vi "主程序.vi"() -> ()   [LabVIEW 2018]
panel:
  out "总用时（s）":dbl
  out "结束时间":u32
  out "开始时间":u32
  out "错误输出":errorcluster
  out "sigma大小5":i32[](array[numeric])
  out "sigma大小4":i32[](array[numeric])
  out "sigma大小3":i32[](array[numeric])
  out "sigma大小2":i32[](array[numeric])
  out "sigma大小1":i32[](array[numeric])
  out "sigma大小":i32[](array[numeric])
  out "cof大小":i32[](array[numeric])
  out "识别结束":bool
  out "最大值":i32
  out "距离":dbl[](array[numeric])
  out "训练完成":bool
  in  "说话人 6 sigma 2":path=path "D:/Desktop/audio/sigma_anjiale3.lvm"
  in  "说话人 6 mu 2":path=path "D:/Desktop/audio/mu_anjiale3.lvm"
  in  "说话人 5 sigma 2":path=path "D:/Desktop/audio/sigma_zhuqiseng3.lvm"
  in  "说话人 5 mu 2":path=path "D:/Desktop/audio/mu_zhuqiseng3.lvm"
  in  "说话人 4 sigma 2":path=path "D:/Desktop/audio/sigma_lianglv3.lvm"
  in  "说话人 4 mu 2":path=path "D:/Desktop/audio/mu_lianglv3.lvm"
  in  "说话人 4 pai 2":path=path "D:/Desktop/audio/pai_lianglv3.lvm"
  in  "说话人 3 sigma 2":path=path "D:/Desktop/audio/sigma_叶雪花.lvm"
  in  "说话人 3 mu 2":path=path "D:/Desktop/audio/mu_叶雪花.lvm"
  in  "说话人 3 pai 2":path=path "D:/Desktop/audio/pai_叶雪花.lvm"
  in  "说话人 2 sigma 2":path=path "D:/Desktop/audio/sigma_赵霞.lvm"
  in  "说话人 2 mu 2":path=path "D:/Desktop/audio/mu_赵霞.lvm"
  in  "说话人 2 pai 2":path=path "D:/Desktop/audio/pai_赵霞.lvm"
  in  "说话人 1 sigma":path=path "D:/Desktop/audio/sigma_胡楠.lvm"
  in  "说话人 1 mu":path=path "D:/Desktop/audio/mu_胡楠.lvm"
  out "提示框":string
  out "滤波后":dbl[](graph)
  out "待识别语音":dbl[](graph)
  in  "说话人 6 pai":path=path "D:/Desktop/audio/pai_anjiale3.lvm"
  in  "说话人 5 pai":path=path "D:/Desktop/audio/pai_zhuqiseng3.lvm"
  in  "说话人 1 pai":path=path "D:/Desktop/audio/pai_胡楠.lvm"
  out "确定的人":string
  out "最大似然距离":dbl format="%.2f"
  in  "语音识别":bool
  in  "语音训练":bool
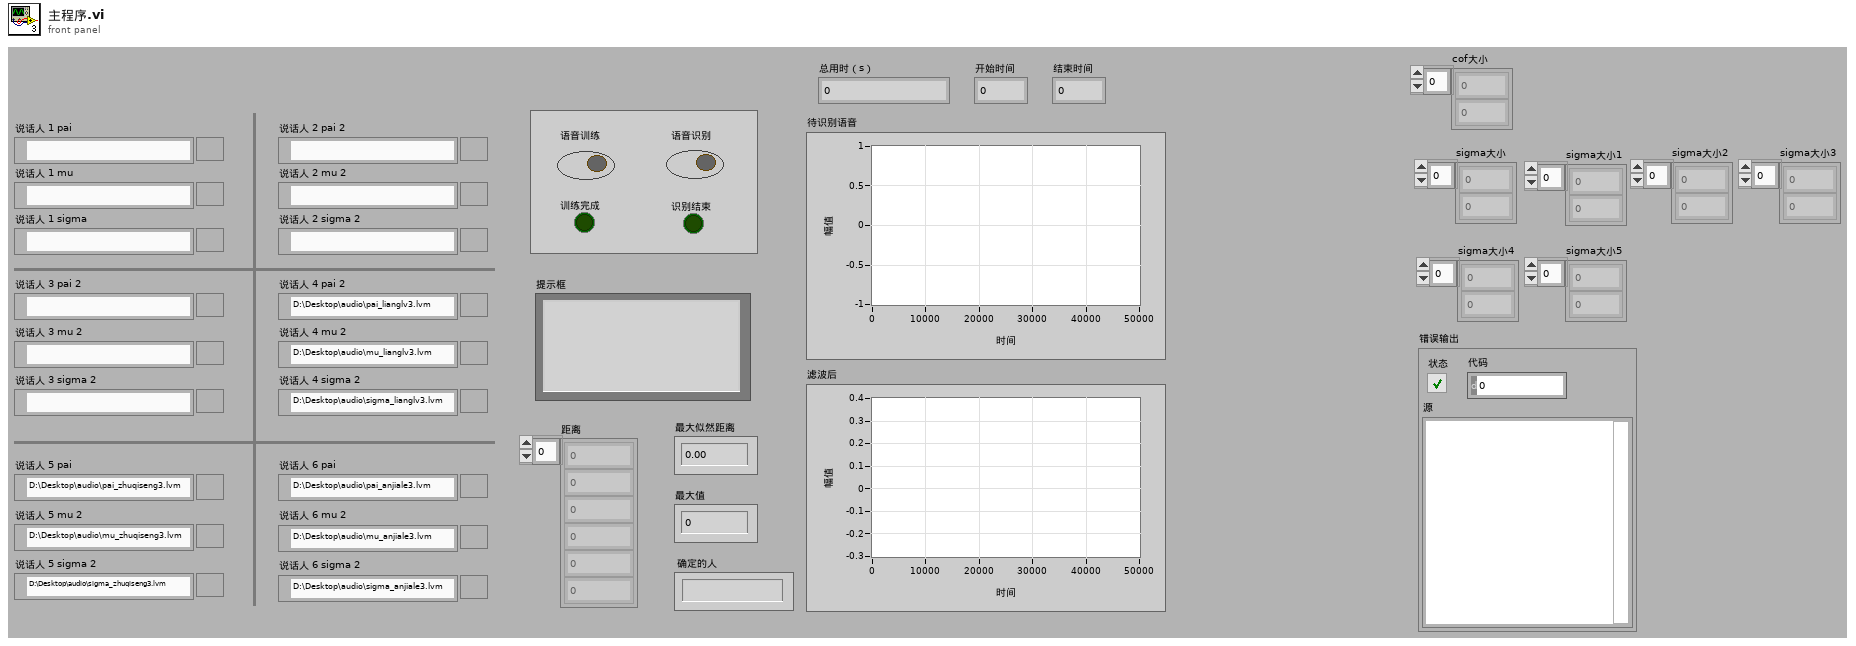
[diagram p1: front panel]
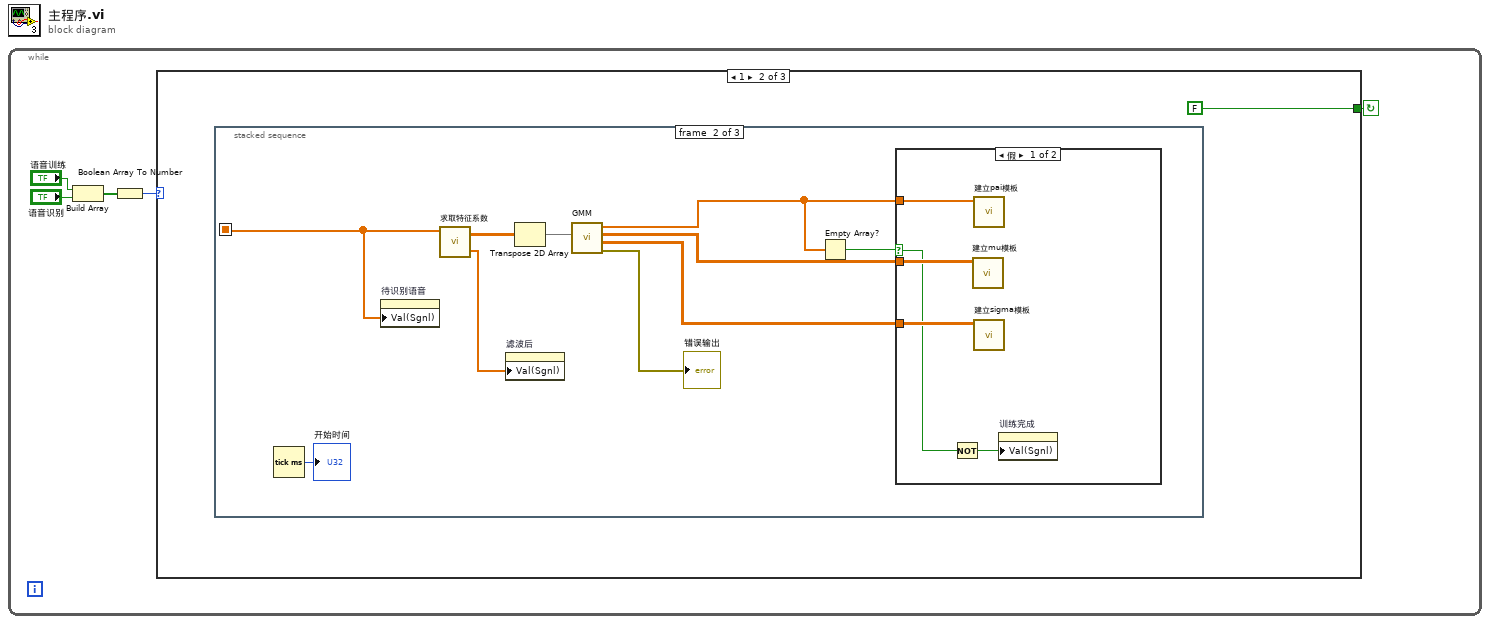
[diagram p0: block diagram]
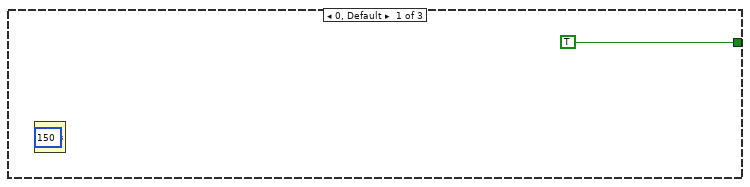
[diagram p2: hidden frame]
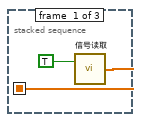
[diagram p3: hidden frame]
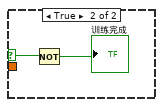
[diagram p4: hidden frame]
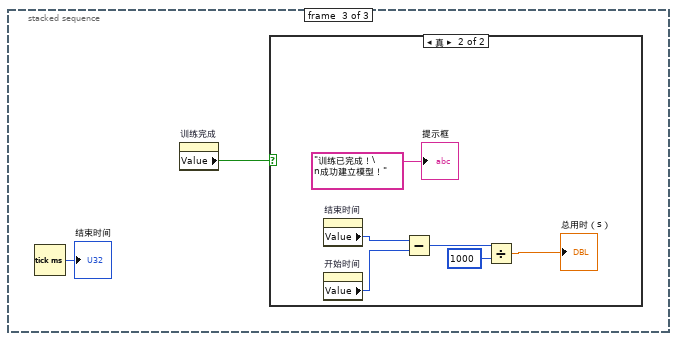
[diagram p5: hidden frame]
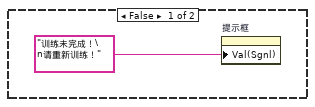
[diagram p6: hidden frame]
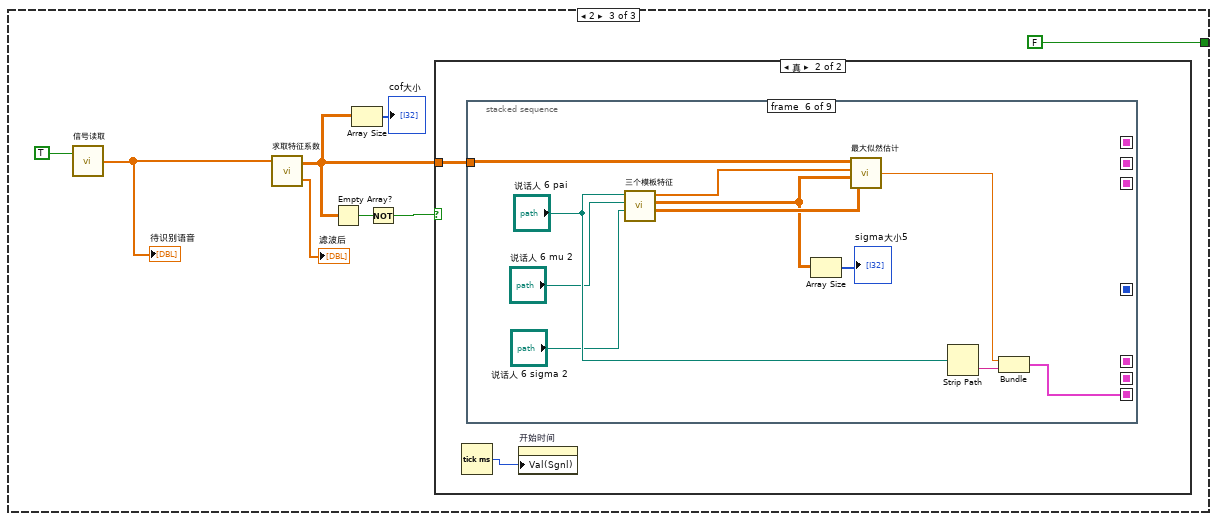
[diagram p7: hidden frame]
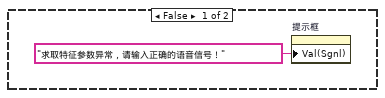
[diagram p8: hidden frame]
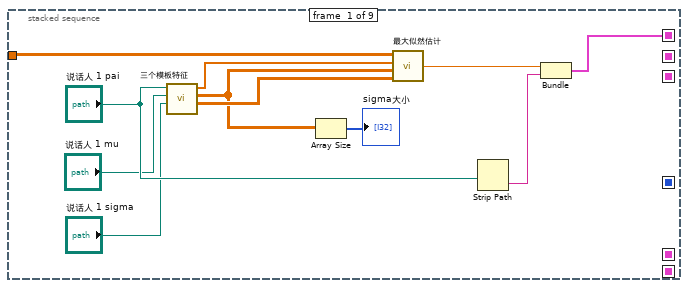
[diagram p9: hidden frame]
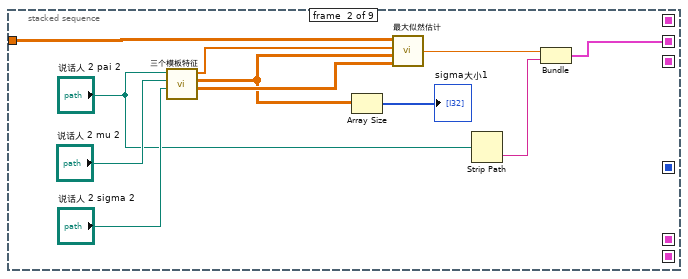
[diagram p10: hidden frame]
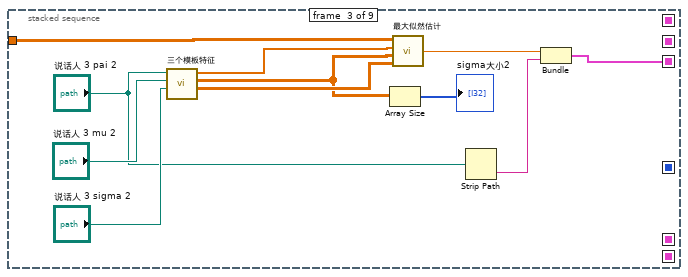
[diagram p11: hidden frame]
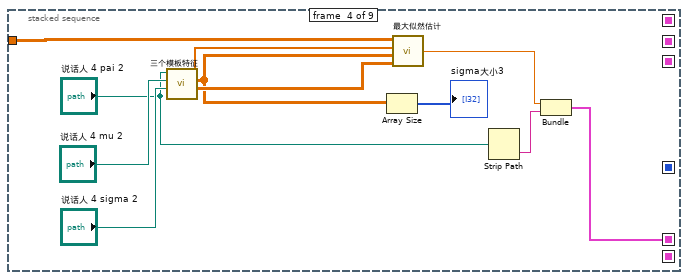
[diagram p12: hidden frame]
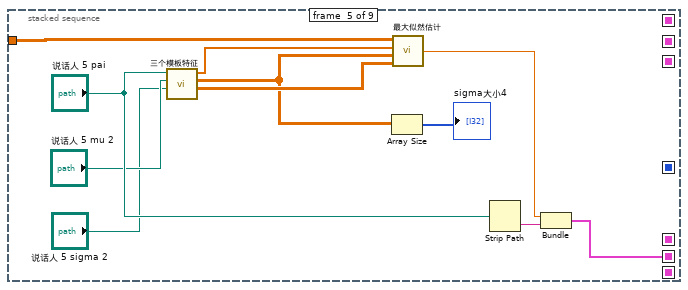
[diagram p13: hidden frame]
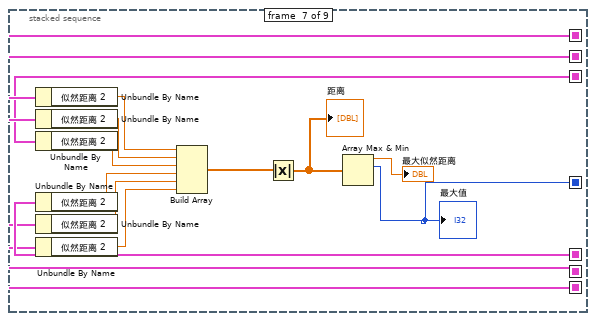
[diagram p14: hidden frame]
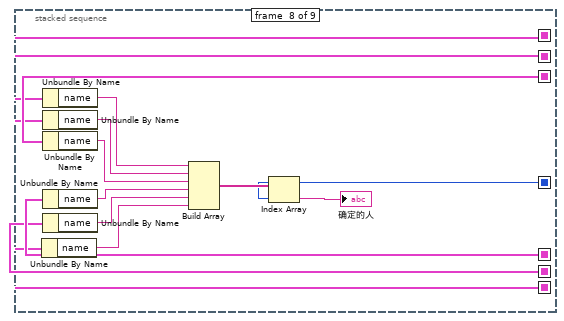
[diagram p15: hidden frame]
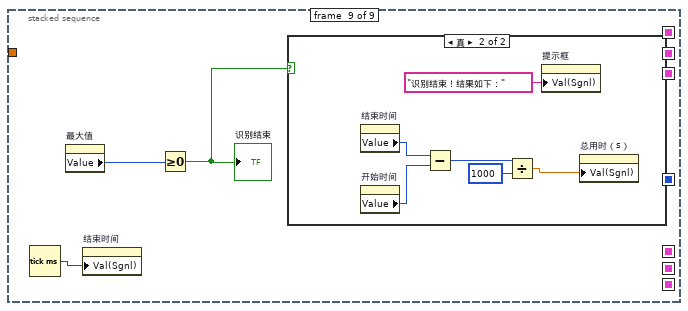
[diagram p16: hidden frame]
diagram:
  n1 = while {
    stop <- w1 continue-if-true
    n2 = Build Array("语音训练", "语音识别") -> (w3:bool[])
    n3 = Boolean Array To Number(Boolean array=w3) -> (number=w2:u32)
    n4 = case shown="1" w2 {
      tunnel: [TRUE FALSE FALSE] -> w1
      frame 0, Default {
        n5 = Wait (ms)(milliseconds to wait=u32 150) -> ()  [unwired: 1 out]
      }
      frame 1 {
        n6 = stacked-sequence {
          seq-local: [w9 _ _] -> [_ w11 _]
          frame #0 {
            n7 = call "信号读取.vi"("Boolean"=TRUE) -> ("mono 16-bit"=w9:dbl[])  [unwired: 1 in]
          }
          frame #1 {
            n8 = Tick Count (ms)() -> (millisecond timer value=→"开始时间":u32)
            n9 = property on="待识别语音" class="WFGraph (严格)"("Val(Sgnl)"=w11) -> ()  [unwired: 2 in, 2 out]
            n10 = call "求取特征系数.vi"("speech"=w11) -> ("波形图"=w16:dbl[], "cof"=w13:dbl[][])  [unwired: 2 in]
            n11 = property on="滤波后" class="WFGraph (严格)"("Val(Sgnl)"=w16) -> ()  [unwired: 2 in, 2 out]
            n12 = Transpose 2D Array(2D array=w13) -> (transposed array=w14:dbl[][])
            n13 = call "GMM.vi"("cof"=w14) -> ("错误输出"=→"错误输出":errorcluster, "sigema"=w20:dbl[][], "mu"=w19:dbl[][], "pai"=w17:dbl[])  [unwired: 6 in]
            n14 = Empty Array?(array=w17) -> (empty?=w18:bool)
            n15 = case shown="假" w18 {
              selector: w18 -> [w22 w27]
              tunnel: w17 -> [w25 _]
              tunnel: w19 -> [w24 _]
              tunnel: w20 -> [w23 _]
              frame False {
                n16 = Not(x=w22) -> (.not. x?=w21:bool)
                n17 = call "建立mu模板.vi"("输入MFCC"=w24) -> ()  [unwired: 11 in]
                n18 = call "建立pai模板.vi"("输入MFCC"=w25) -> ()  [unwired: 11 in]
                n19 = call "建立sigma模板.vi"("输入MFCC"=w23) -> ()  [unwired: 11 in]
                n20 = property on="训练完成" class="Bool (严格)"("Val(Sgnl)"=w21) -> ()  [unwired: 2 in, 2 out]
              }
              frame True {
                n21 = Not(x=w27) -> (.not. x?=→"训练完成":bool)
              }
            }
          }
          frame #2 {
            n22 = Tick Count (ms)() -> (millisecond timer value=→"结束时间":u32)
            n23 = property on="训练完成" class="Bool (严格)"() -> ("Value"=w29:bool)  [unwired: 2 in, 2 out]
            n24 = case shown="真" w29 {
              frame False {
                n25 = property on="提示框" class="Str"("Val(Sgnl)"="训练未完成！\n请重新训练！") -> ()  [unwired: 2 in, 2 out]
              }
              frame True {
                n26 = property on="结束时间" class="DigNum (严格)"() -> ("Value"=w32:u32)  [unwired: 2 in, 2 out]
                n27 = property on="开始时间" class="DigNum (严格)"() -> ("Value"=w31:u32)  [unwired: 2 in, 2 out]
                n28 = Subtract(x=w32, y=w31) -> (x-y=w34:u32)
                n29 = Divide(x=w34, y=u32 1000) -> (x/y=→"总用时（s）":dbl)
                "提示框" <- "训练已完成！\n成功建立模型！"
              }
            }
          }
        }
      }
      frame 2 {
        n30 = call "信号读取.vi"("Boolean"=TRUE) -> ("mono 16-bit"=w39:dbl[])  [unwired: 1 in]
        "待识别语音" <- w39
        n31 = call "求取特征系数.vi"("speech"=w39) -> ("波形图"=→"滤波后":dbl[], "cof"=w38:dbl[][])  [unwired: 2 in]
        n32 = Empty Array?(array=w38) -> (empty?=w43:bool)
        n33 = Array Size(array=w38) -> (size(s)=→"cof大小":i32[])
        n34 = Not(x=w43) -> (.not. x?=w42:bool)
        n35 = case shown="真" w42 {
          tunnel: w38 -> [_ w47]
          frame False {
            n36 = property on="提示框" class="Str"("Val(Sgnl)"="求取特征参数异常，请输入正确的语音信号！" ("值(信号)")) -> ()  [unwired: 2 in, 2 out]
          }
          frame True {
            n37 = Tick Count (ms)() -> (millisecond timer value=w46:u32)
            n38 = stacked-sequence {
              seq-local: [_ _ _ _ _ _ w115 _ _] -> [_ _ _ _ _ _ _ w137 _]
              seq-local: [w57 _ _ _ _ _ _ _ _] -> [_ _ _ _ _ _ w129 w134 _]
              seq-local: [_ w68 _ _ _ _ _ _ _] -> [_ _ _ _ _ _ w128 w135 _]
              seq-local: [_ _ w79 _ _ _ _ _ _] -> [_ _ _ _ _ _ w127 w136 _]
              seq-local: [_ _ _ w90 _ _ _ _ _] -> [_ _ _ _ _ _ w126 w133 _]
              seq-local: [_ _ _ _ w101 _ _ _ _] -> [_ _ _ _ _ _ w125 w132 _]
              seq-local: [_ _ _ _ _ w112 _ _ _] -> [_ _ _ _ _ _ w124 w131 _]
              tunnel: w47 -> [w51 w65 w77 w88 w98 w109 _ _ _]
              frame #0 {
                n39 = call "三个模板特征.vi"("Filename 3"="说话人 1 sigma", "Filename 2"="说话人 1 mu", "Filename"="说话人 1 pai") -> ("sigma 4"=w49:dbl[][], "mu 3"=w48:dbl[][], "pai 2"=w54:dbl[])  [unwired: 5 in]
                n40 = Array Size(array=w48) -> (size(s)=→"sigma大小":i32[])
                n41 = call "最大似然估计.vi"("sigma"=w49, "mu"=w48, "pai"=w54, "cof"=w51) -> ("似然距离 2"=w55:dbl)
                n42 = Strip Path(path="说话人 1 pai") -> (name=w58:string)  [unwired: 1 out]
                n43 = Bundle("似然距离 2"=w55, "name"=w58) -> (w57:cluster{"似然距离 2":dbl, "name":string})  [unwired: 1 in]
              }
              frame #1 {
                n44 = call "三个模板特征.vi"("Filename 3"="说话人 2 sigma 2", "Filename 2"="说话人 2 mu 2", "Filename"="说话人 2 pai 2") -> ("sigma 4"=w61:dbl[][], "mu 3"=w59:dbl[][], "pai 2"=w67:dbl[])  [unwired: 5 in]
                n45 = Array Size(array=w59) -> (size(s)=→"sigma大小1":i32[])
                n46 = call "最大似然估计.vi"("sigma"=w61, "mu"=w59, "pai"=w67, "cof"=w65) -> ("似然距离 2"=w66:dbl)
                n47 = Strip Path(path="说话人 2 pai 2") -> (name=w69:string)  [unwired: 1 out]
                n48 = Bundle("似然距离 2"=w66, "name"=w69) -> (w68:cluster{"似然距离 2":dbl, "name":string})  [unwired: 1 in]
              }
              frame #2 {
                n49 = call "三个模板特征.vi"("Filename 3"="说话人 3 sigma 2", "Filename 2"="说话人 3 mu 2", "Filename"="说话人 3 pai 2") -> ("sigma 4"=w72:dbl[][], "mu 3"=w70:dbl[][], "pai 2"=w78:dbl[])  [unwired: 5 in]
                n50 = Array Size(array=w70) -> (size(s)=→"sigma大小2":i32[])
                n51 = call "最大似然估计.vi"("sigma"=w72, "mu"=w70, "pai"=w78, "cof"=w77) -> ("似然距离 2"=w76:dbl)
                n52 = Strip Path(path="说话人 3 pai 2") -> (name=w80:string)  [unwired: 1 out]
                n53 = Bundle("似然距离 2"=w76, "name"=w80) -> (w79:cluster{"似然距离 2":dbl, "name":string})  [unwired: 1 in]
              }
              frame #3 {
                n54 = call "三个模板特征.vi"("Filename 3"="说话人 4 sigma 2", "Filename 2"="说话人 4 mu 2", "Filename"="说话人 4 pai 2") -> ("sigma 4"=w83:dbl[][], "mu 3"=w81:dbl[][], "pai 2"=w87:dbl[])  [unwired: 5 in]
                n55 = Array Size(array=w81) -> (size(s)=→"sigma大小3":i32[])
                n56 = call "最大似然估计.vi"("sigma"=w83, "mu"=w81, "pai"=w87, "cof"=w88) -> ("似然距离 2"=w89:dbl)
                n57 = Strip Path(path="说话人 4 pai 2") -> (name=w91:string)  [unwired: 1 out]
                n58 = Bundle("似然距离 2"=w89, "name"=w91) -> (w90:cluster{"似然距离 2":dbl, "name":string})  [unwired: 1 in]
              }
              frame #4 {
                n59 = call "三个模板特征.vi"("Filename 3"="说话人 5 sigma 2", "Filename 2"="说话人 5 mu 2", "Filename"="说话人 5 pai") -> ("sigma 4"=w94:dbl[][], "mu 3"=w92:dbl[][], "pai 2"=w97:dbl[])  [unwired: 5 in]
                n60 = Array Size(array=w92) -> (size(s)=→"sigma大小4":i32[])
                n61 = call "最大似然估计.vi"("sigma"=w94, "mu"=w92, "pai"=w97, "cof"=w98) -> ("似然距离 2"=w99:dbl)
                n62 = Strip Path(path="说话人 5 pai") -> (name=w102:string)  [unwired: 1 out]
                n63 = Bundle("似然距离 2"=w99, "name"=w102) -> (w101:cluster{"似然距离 2":dbl, "name":string})  [unwired: 1 in]
              }
              frame #5 {
                n64 = call "三个模板特征.vi"("Filename 3"="说话人 6 sigma 2", "Filename 2"="说话人 6 mu 2", "Filename"="说话人 6 pai") -> ("sigma 4"=w107:dbl[][], "mu 3"=w104:dbl[][], "pai 2"=w108:dbl[])  [unwired: 5 in]
                n65 = Array Size(array=w104) -> (size(s)=→"sigma大小5":i32[])
                n66 = call "最大似然估计.vi"("sigma"=w107, "mu"=w104, "pai"=w108, "cof"=w109) -> ("似然距离 2"=w110:dbl)
                n67 = Strip Path(path="说话人 6 pai") -> (name=w113:string)  [unwired: 1 out]
                n68 = Bundle("似然距离 2"=w110, "name"=w113) -> (w112:cluster{"似然距离 2":dbl, "name":string})  [unwired: 1 in]
              }
              frame #6 {
                n69 = Unbundle By Name(w129) -> ("似然距离 2"=w123:dbl)
                n70 = Unbundle By Name(w128) -> ("似然距离 2"=w122:dbl)
                n71 = Unbundle By Name(w127) -> ("似然距离 2"=w121:dbl)
                n72 = Unbundle By Name(w126) -> ("似然距离 2"=w120:dbl)
                n73 = Unbundle By Name(w125) -> ("似然距离 2"=w119:dbl)
                n74 = Unbundle By Name(w124) -> ("似然距离 2"=w118:dbl)
                n75 = Build Array(w123, w122, w121, w120, w119, w118) -> (w116:dbl[])
                n76 = Absolute Value(x=w116) -> (abs(x)=w117:dbl[])
                "距离" <- w117
                n77 = Array Max & Min(array=w117) -> (max value=→"最大似然距离":dbl, max index (indices)=w115:i32)  [unwired: 2 out]
                "最大值" <- w115
              }
              frame #7 {
                n78 = Unbundle By Name(w131) -> ("name"=w138:string)
                n79 = Unbundle By Name(w134) -> ("name"=w143:string)
                n80 = Unbundle By Name(w135) -> ("name"=w142:string)
                n81 = Unbundle By Name(w136) -> ("name"=w141:string)
                n82 = Unbundle By Name(w133) -> ("name"=w140:string)
                n83 = Unbundle By Name(w132) -> ("name"=w139:string)
                n84 = Build Array(w143, w142, w141, w140, w139, w138) -> (w144:string[])
                n85 = Index Array(array=w144, index=w137) -> (element=→"确定的人":string)
              }
              frame #8 {
                n86 = Tick Count (ms)() -> (millisecond timer value=w145:u32)
                n87 = property on="最大值" class="DigNum (严格)"() -> ("Value"=w147:i32)  [unwired: 2 in, 2 out]
                n88 = property on="结束时间" class="DigNum (严格)"("Val(Sgnl)"=w145) -> ()  [unwired: 2 in, 2 out]
                n89 = Greater Or Equal To 0?(x=w147) -> (x >= 0?=w146:bool)
                "识别结束" <- w146
                n90 = case shown="真" w146 {
                  frame False {
                  }
                  frame True {
                    n91 = property on="结束时间" class="DigNum (严格)"() -> ("Value"=w149:u32)  [unwired: 2 in, 2 out]
                    n92 = property on="开始时间" class="DigNum (严格)"() -> ("Value"=w148:u32)  [unwired: 2 in, 2 out]
                    n93 = Subtract(x=w149, y=w148) -> (x-y=w152:u32)
                    n94 = Divide(x=w152, y=u32 1000) -> (x/y=w150:dbl)
                    n95 = property on="提示框" class="Str"("Val(Sgnl)"="识别结束！结果如下：" ("值(信号)")) -> ()  [unwired: 2 in, 2 out]
                    n96 = property on="总用时（s）" class="DigNum (严格)"("Val(Sgnl)"=w150) -> ()  [unwired: 2 in, 2 out]
                  }
                }
              }
            }
            n97 = property on="开始时间" class="DigNum (严格)"("Val(Sgnl)"=w46) -> ()  [unwired: 2 in, 2 out]
          }
        }
      }
    }
  }
